vi "SVL Max-Min Level (1 Ch).vi"(6 "restart averaging (F)":bool, 8 "error in (no error)":errorcluster, 11 "scaled signal [EU]":waveform(dbl)) -> (0 "error out":errorcluster, 2 "unit label":string, 3 "max-min level [EU]":dbl=nan format="%.2f", 5 "min level [EU]":dbl=nan format="%.2f", 7 "max level [EU]":dbl=nan format="%.2f")   [LabVIEW 2017, in "SoundVib_VibrationLevel.lvlib"]
doc: "Computes the maximum and minimum levels of all previous values and the difference between the maximum and minimum levels of <B>scaled signal [EU]</B> or <B>even-angle signal [EU]</B>. <B>scaled signal [EU]</B> should have a zero DC component. You can attenuate the DC component with hardware AC-coupling filters and with software high-pass filters. Wire data to the <B>scaled signal [EU]</B> input to determine the polymorphic instance to use or manually select the instance."
uses:
  <vilib>/addons/Sound and Vibration/svt_Level/SoundVib_VibrationLevel.lvlib
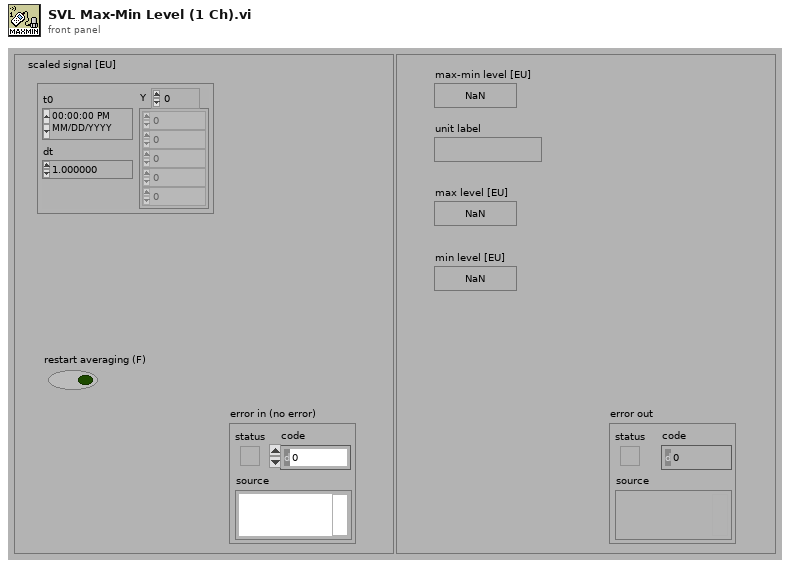
[diagram p1: front panel]
types:
  T1 = enum16{"RMS", "Running RMS", "Exp avg  ", "Dec exp avg ", "Peak", "Crest"}
  T2 = enum16{"Reset filter", "Restart averaging", "Continue processing"}
  T3 = typedef "svc_Channel Info.ctl" = cluster{"sensor sensitivity":dbl, "engineering units":T4, "dB reference":dbl, "custom label":string, "weighting filter":T5, "pregain":dbl}
  T4 = typedef "svc_Engineering Units Text Ring.ctl" = u16
  T5 = typedef "svc_Weighting Filter Text Ring.ctl" = u16
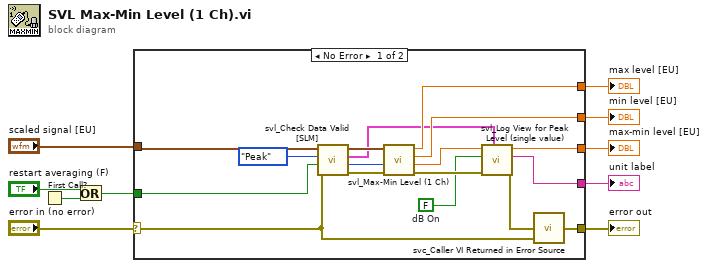
[diagram p0: block diagram]
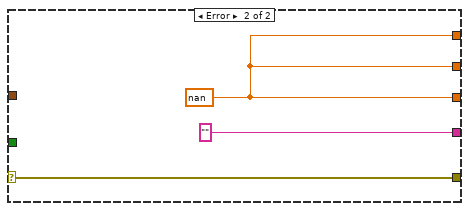
[diagram p2: hidden frame]
diagram:
  n1 = First Call?() -> (First Call?: T/F=w5:bool)
  n2 = Or(x="restart averaging (F)", y=w5) -> (x .or. y?=w3:bool)
  n3 = case shown="No Error" "error in (no error)" {
    tunnel: [w25 w28] -> w8
    tunnel: [w24 "" ("unit label")] -> w7
    tunnel: "scaled signal [EU]" -> [w13 _]
    tunnel: w3 -> [w20 _]
    selector: "error in (no error)" -> [w11 w30]
    tunnel: [w26 w30] -> w10
    tunnel: [w18 w28] -> w2
    tunnel: [w17 w28] -> w1
    frame No Error {
      w15 = FALSE  # dB On
      n4 = call <vilib>:"svl_Check Data Valid [SLM].vi"("error in (no error)"=w11, "restart averaging (F)"=w20, "Level Analysis"=T1."Peak", "scaled signal [EU]"=w13) -> ("error out"=w22:errorcluster, "processing state"=w21:T2, "channel info"=w12:T3, "dup scaled signal [EU]"=w14:waveform(dbl))  [unwired: 4 in]
      n5 = call <vilib>:"svl_Max-Min Level (1 Ch).vi"("error in (no error)"=w22, "processing state"=w21, "scaled signal"=w14) -> ("error out"=w23:errorcluster, "max-min level"=w16:dbl, "final min level"=w17:dbl, "final max level"=w18:dbl)  [unwired: 5 in]
      n6 = call <vilib>:"svl_Log View for Peak Level (single value).vi"("channel info"=w12, "error in (no error)"=w23, "dB On (T)"=w15, "peak level [EU]"=w16) -> ("error out"=w27:errorcluster, "unit label"=w24:string, "peak level [EU]"=w25:dbl)  [unwired: 5 in]
      n7 = call <vilib>:"svc_Caller VI Returned in Error Source.vi"("warning input to caller"=w11, "error in (no error)"=w27) -> ("error out"=w26:errorcluster)  [unwired: 3 in]
    }
    frame Error {
      w28 = nan ("energy level [EU^2 rms]")
    }
  }
  "max-min level [EU]" <- w8
  "unit label" <- w7
  "error out" <- w10
  "max level [EU]" <- w2
  "min level [EU]" <- w1
